vi "Yscaling_FBL.vi"(6 "Scaling?":bool, 8 "Nano Z Read":dbl, 9 "Current Maxed?":bool, 10 "Y":dbl, 11 "Plane Height":dbl) -> (3 "y scaled (m)":dbl, 4 "Zpos Graph (nm)":cluster{dbl, "function return":dbl})   [LabVIEW 2019]
uses:
  GlobalClicksHeight_FBL.vi
  <userlib>/HapticSTM/HapticSTM.lvlib
panel:
  out "Testoutput":dbl
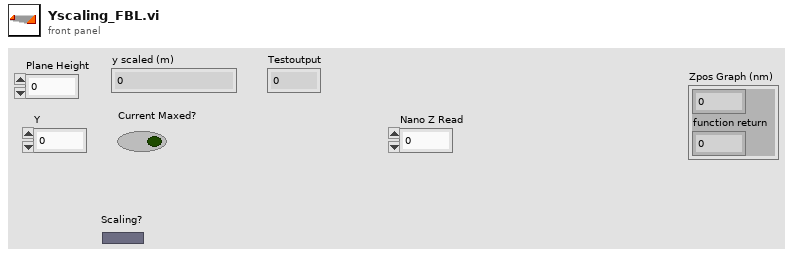
[diagram p1: front panel]
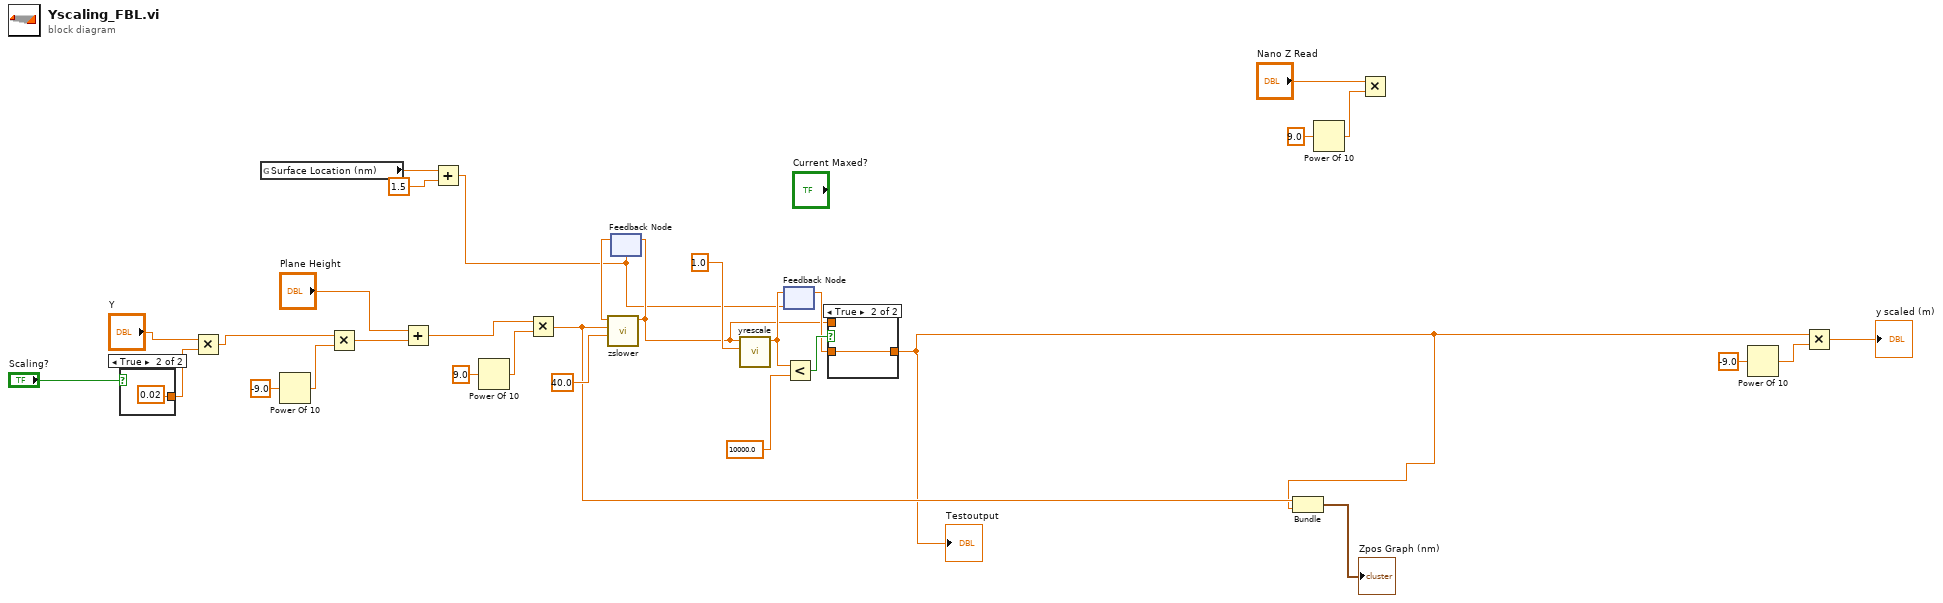
[diagram p0: block diagram]
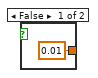
[diagram p2: hidden frame]
diagram:
  n1 = case shown="True" "Scaling?" {
    tunnel: [0.01 ("y") 0.02 ("y")] -> w2
    frame False {
    }
    frame True {
    }
  }
  n2 = Multiply(x="Y", y=w2) -> (x*y=w27:dbl)
  n3 = global read "GlobalClicksHeight_FBL.vi" "Surface Location (nm)"() -> (w5:dbl)
  n4 = Power Of 10(x=-9.0) -> (10^x=w26:dbl)
  n5 = Multiply(x=w27, y=w26) -> (x*y=w28:dbl)
  n6 = Add(x="Plane Height", y=w28) -> (x+y=w31:dbl)
  n7 = Add(x=w5, y=1.5) -> (x+y=w4:dbl)
  n8 = Power Of 10(x=9.0) -> (10^x=w30:dbl)
  n9 = Multiply(x=w31, y=w30) -> (x*y=w9:dbl)
  n10 = feedback #1(w4) -> (w11:dbl)
  n11 = call <userlib>:"zslower.vi"("maxvel"=40.0, "labview_zpos_write"=w9, "nanonis_zpos_read"=w11) -> ("function return"=w7:dbl)  [unwired: 8 in]
  n12 = feedback-in #1(w7) -> ()
  n13 = call <userlib>:"yrescale.vi"("scalingfactor"=1.0, "ylabview"=w7) -> ("function return"=w8:dbl)  [unwired: 9 in]
  n14 = feedback-in #2(w8) -> ()
  n15 = feedback #2(w4) -> (w16:dbl)
  n16 = Less?(x=w8, y=10000.0) -> (x < y?=w17:bool)
  n17 = case shown="True" w17 {
    tunnel: [w34 w35] -> w1
    tunnel: w16 -> [_ w35]
    tunnel: w7 -> [w34 _]
    frame False {
    }
    frame True {
    }
  }
  "Testoutput" <- w1
  n18 = Bundle(w9, "function return"=w1) -> (→"Zpos Graph (nm)":cluster{dbl, "function return":dbl})  [unwired: 1 in]
  n19 = Power Of 10(x=9.0) -> (10^x=w15:dbl)
  n20 = Multiply(x="Nano Z Read", y=w15) -> ()  [unwired: 1 out]
  n21 = Power Of 10(x=-9.0) -> (10^x=w21:dbl)
  n22 = Multiply(x=w1, y=w21) -> (x*y=→"y scaled (m)":dbl)
